vi "Close Framework Event Log.vi"(8 "error in (no error)":errorcluster, 10 "Deferred Close Time (3000 ms)":u32, 11 "IObserver in":refnum<class "IObserver.lvclass">) -> ()   [LabVIEW 2017, in "IObserver.lvlib" / "IObserver.lvclass"]
uses:
  IObserver.lvclass
  IObserver.lvclass/IObserver.ctl
  gpm_packages/@cs/event-logger/Source/Composed Log/LoggerReference/LoggerReference.lvclass
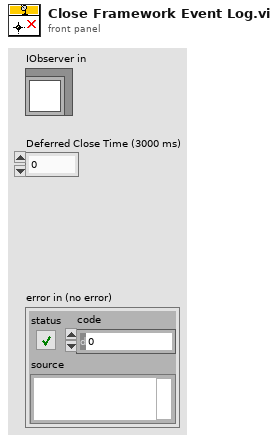
[diagram p1: front panel]
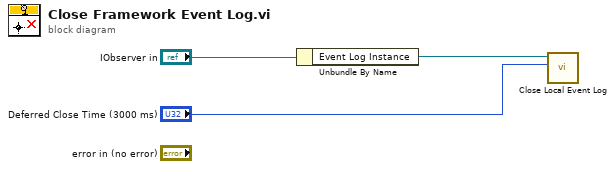
[diagram p0: block diagram]
diagram:
  n1 = Unbundle By Name("IObserver in") -> ("Event Log Instance"=w2:refnum<class "LoggerReference.lvclass">)
  n2 = call "Close Local Event Log.vi"("Deferred Close Time (0 ms)"="Deferred Close Time (3000 ms)", "Log Instance"=w2) -> ()  [unwired: 9 in, 1 out]
